vi "FUNCT+MAP.vi"(7 "mode":u8, 9 "Funct Map":cluster{"In":u8, "Out":u8}={"In"=22, "Out"=0} {"In" items=["ABSOLUTE"=16, "RELATIVE"=8, "DISCRETE"=4]}, 11 "Python in":string="import machine, utime\n\ntx = machine.Pin('Y9', machine.Pin.OUT)\nrx = machine.Pin('Y10', machine.Pin.IN)\ntx.value(b'\\x00')\nutime.sleep_ms(500)\ntx.value(1)\n\nuart = machine.UART(3)\nuart.init(baudrate=2400, bits=8, parity=None, stop=1)\n\nuart.write(0)\nuart.write(b'\\x40\\x23\\x9C')\nuart.write(b'\\x98\\x00\\x4C\\x69\\x67\\x68\\x74\\x00\\x00\\x00\\x39')\n") -> (3 "Python out":string="import machine, utime\n\ntx = machine.Pin('Y9', machine.Pin.OUT)\nrx = machine.Pin('Y10', machine.Pin.IN)\ntx.value(b'\\x00')\nutime.sleep_ms(500)\ntx.value(1)\n\nuart = machine.UART(3)\nuart.init(baudrate=2400, bits=8, parity=None, stop=1)\n\nuart.write(0)\nuart.write(b'\\x40\\x23\\x9C')\nuart.write(b'\\x98\\x00\\x4C\\x69\\x67\\x68\\x74\\x00\\x00\\x00\\x39')\nuart.write(b'\\x90\\x80\\x01\\x00\\x03\\x00\\xED')\n")   [LabVIEW 2019]
panel:
  out "bytes added":u8[](array[numeric])=[144, 128, 1, 0, 3, 0, 237] format="%.0x"
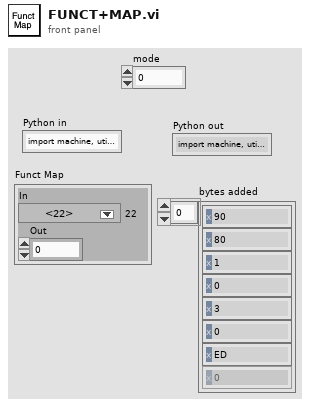
[diagram p1: front panel]
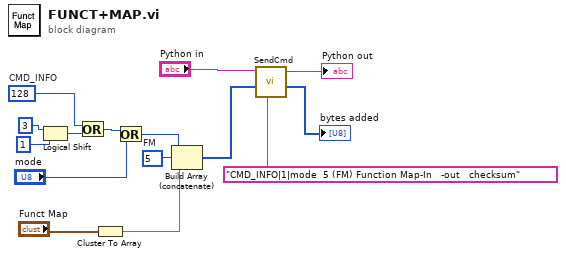
[diagram p0: block diagram]
diagram:
  w2 = u8 5  # FM
  w11 = u8 128  # CMD_INFO
  n1 = Logical Shift(y=i16 3, x=u8 1) -> (x << y=w10:u8)
  n2 = Or(x=w11, y=w10) -> (x .or. y?=w12:u8)
  n3 = Cluster To Array(cluster="Funct Map") -> (array=w5:u8[])
  n4 = Or(x=w12, y="mode") -> (x .or. y?=w3:u8)
  n5 = Build Array (concatenate)(w3, w2, w5) -> (w4:u8[])
  n6 = call <userlib>:"SendCmd.vi"("Comment"="CMD_INFO|1|mode  5 (FM) Function Map-In   -out   checksum", "Array In"=w4, "Python in"="Python in") -> ("Array Sent"=→"bytes added":u8[], "Python out"=→"Python out":string)  [unwired: 7 in]
